vi "Find In Project Recursively.vi"(10 "File":path, 11 "Project Items":refnum<vi>[](array[refnum])) -> (3 "ProjectItem out":refnum<vi>)   [LabVIEW 2020, in "Mock Class Updater.lvclass"]
uses:
  Mock Class Updater.lvclass
  Mock Class Updater.lvclass/Mock Class Updater.ctl
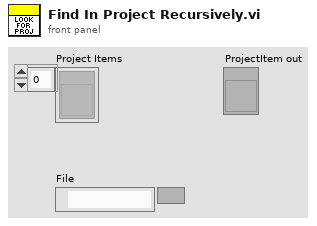
[diagram p1: front panel]
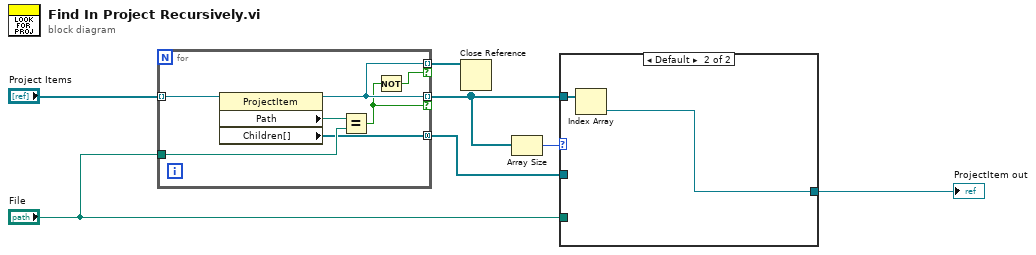
[diagram p0: block diagram]
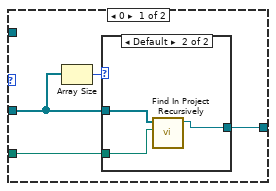
[diagram p2: hidden frame]
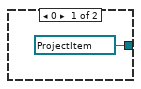
[diagram p3: hidden frame]
diagram:
  n1 = for {
    tunnel: "Project Items" -> [w14] mode=indexing
    tunnel: "File" -> [w12]
    tunnel: [w11] -> w4 mode=indexing if=w10
    tunnel: [w11] -> w5 mode=indexing if=w9
    tunnel: [w8] -> w2 mode=concatenating
    n2 = property class="ProjectItem"(reference=w14) -> (reference out=w11:refnum<vi>, "Path"=w13:path, "Children[]"=w8:refnum<vi>[])  [unwired: 1 in, 1 out]
    n3 = Equal?(x=w13, y=w12) -> (x = y?=w10:bool)
    n4 = Not(x=w10) -> (.not. x?=w9:bool)
  }
  n5 = Close Reference(reference=w5) -> ()  [unwired: 1 in, 1 out]
  n6 = Array Size(array=w4) -> (size(s)=w3:i32)
  n7 = case shown="Default" w3 {
    tunnel: [w17 w24] -> w7
    tunnel: w4 -> [_ w23]
    tunnel: w2 -> [w16 _]
    tunnel: "File" -> [w18 _]
    frame 0 {
      n8 = Array Size(array=w16) -> (size(s)=w15:i32)
      n9 = case shown="Default" w15 {
        tunnel: w18 -> [_ w22]
        tunnel: [refnum<vi> refnum ("ProjectItem out") w21] -> w17
        tunnel: w16 -> [_ w20]
        frame 0 {
        }
        frame Default {
          n10 = call "Find In Project Recursively.vi"("File"=w22, "Project Items"=w20) -> ("ProjectItem out"=w21:refnum<vi>)  [unwired: 9 in]
        }
      }
    }
    frame Default {
      n11 = Index Array(array=w23) -> (element=w24:refnum<vi>)  [unwired: 1 in]
    }
  }
  "ProjectItem out" <- w7
